vi "Measurement - PAE.vi"(7 "measure call context in":refnum<class "Measure Call Context.lvclass">, 8 "error in":errorcluster, 9 "RFmx Settings":T1={"RFmx Name"="5842_0", "RFmx Port"="", "Attenuation"={"Mode"=enum."Constant Attenuation", "Constant Attenuation"={"RFmx External Attenuation (dB)"=1.2}, "s2p File"={"RFmx S-Parameters Orientation"=24000, "RFmx Attenuation s2p File"=path ""}}} {"Attenuation"."s2p File"."RFmx S-Parameters Orientation" items=["Port1 Towards DUT"=24000, "Port2 Towards DUT"=24001]; "Attenuation"."Constant Attenuation"."RFmx External Attenuation (dB)" format="%.2f"}, 10 "RFSG Settings":T2={"RFSG Name"="5842_0", "RFSG Port"="", "Attenuation"={"Mode"=enum."Constant Attenuation", "Contant Attenuation"={"RFSG External Attenuation (dB)"=2.0}, "s2p File"={"RFSG S-parameters Orientation"=24000, "RFSG s2p File Path"=path ""}}} {"Attenuation"."s2p File"."RFSG S-parameters Orientation" items=["Port1 Towards DUT"=24000, "Port2 Towards DUT"=24001]; "Attenuation"."Contant Attenuation"."RFSG External Attenuation (dB)" format="%.2f"}, 11 "PAE Reference in":T3) -> (0 "error out":errorcluster, 3 "PAE Reference out":T3)   [LabVIEW 2023]
uses:
  <vilib>/niPAEML/Typedefs/Session Handle.ctl
  <vilib>/niPAEML/PAE Reference.lvclass
  Controls/RFSG Config - Compression.ctl
  Controls/RFmx Config - Compression.ctl
  <vilib>/Plug-In SDKs/Measurements/Measure Call Context/Measure Call Context.lvclass
  <instrlib>/niDCPower/nidcpower.llb/niDCPower Wait For Event - Event.ctl
  <vilib>/niPAEML/PAE Reference.lvclass/PAE Reference.ctl
  <vilib>/niPAEML/Accessors/Read RFSG Stimulus Mode.vi
  <vilib>/Analysis/baseanly.llb/Mean (DBL).vi
  <vilib>/RFmx/SpecAn/mx/RFmxSpecAn.llb/RFmxSpecAn TXP Fetch Measurement.vi
  <resource>/objmgr/RFmxSpecAn.rc
  <vilib>/niPAEML/PAE Measurement.lvlib
  <vilib>/Analysis/NI_AALBase.lvlib
panel:
  out "Current":dbl[](graph)
  out "Voltage":dbl[](graph)
  out "Pout":dbl[](graph)
  out "RF Input Sweep":dbl[](graph)
  out "Frequency Sweep":dbl[](graph)
  out "Power  Sweep Progress":dbl(slide)=1.0 scale=0.0..1.0
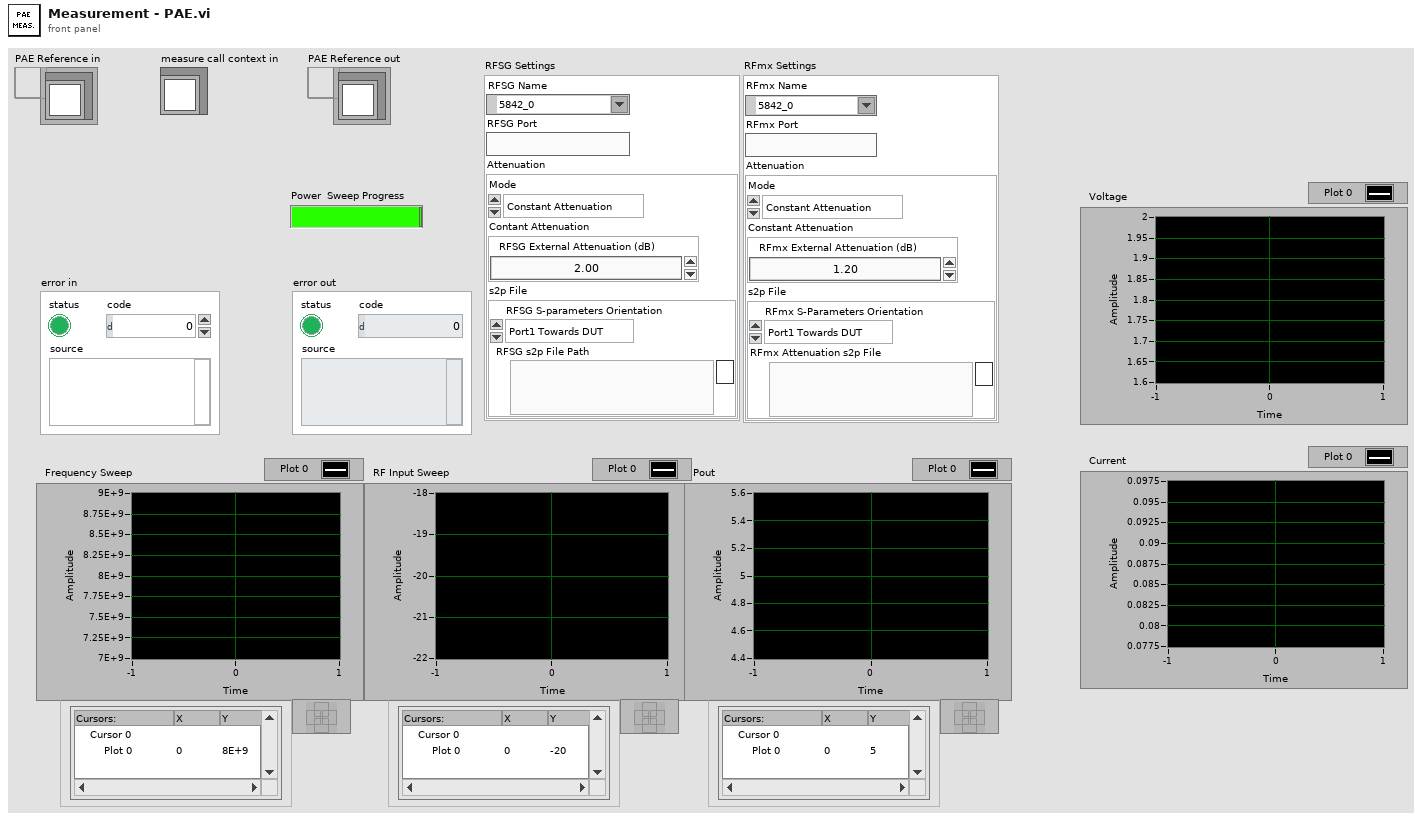
[diagram p1: front panel]
types:
  T1 = typedef "RFmx Config - Compression.ctl" = cluster{"RFmx Name":refnum<k15>, "RFmx Port":string, "Attenuation":cluster{"Mode":enum32{"<None>", "Constant Attenuation", "s2p File"}, "Constant Attenuation":cluster{"RFmx External Attenuation (dB)":dbl}, "s2p File":cluster{"RFmx S-Parameters Orientation":i32, "RFmx Attenuation s2p File":path}}}
  T2 = typedef "RFSG Config - Compression.ctl" = cluster{"RFSG Name":refnum<k15>, "RFSG Port":string, "Attenuation":cluster{"Mode":enum32{"<None>", "Constant Attenuation", "s2p File"}, "Contant Attenuation":cluster{"RFSG External Attenuation (dB)":dbl}, "s2p File":cluster{"RFSG S-parameters Orientation":i32, "RFSG s2p File Path":path}}}
  T3 = typedef "PAE Measurement.lvlib/PAE Reference.lvclass/Session Handle.ctl" = refnum<data-value>
  T4 = enum32{"<None>", "Constant Attenuation", "s2p File"}
  T5 = typedef "niDCPower Wait For Event - Event.ctl" = i32
  T6 = typedef "PAE Measurement.lvlib/PAE Reference.lvclass/RFSG Stimulus Mode.ctl" = enum16{"CW", "Pulsed CW"}
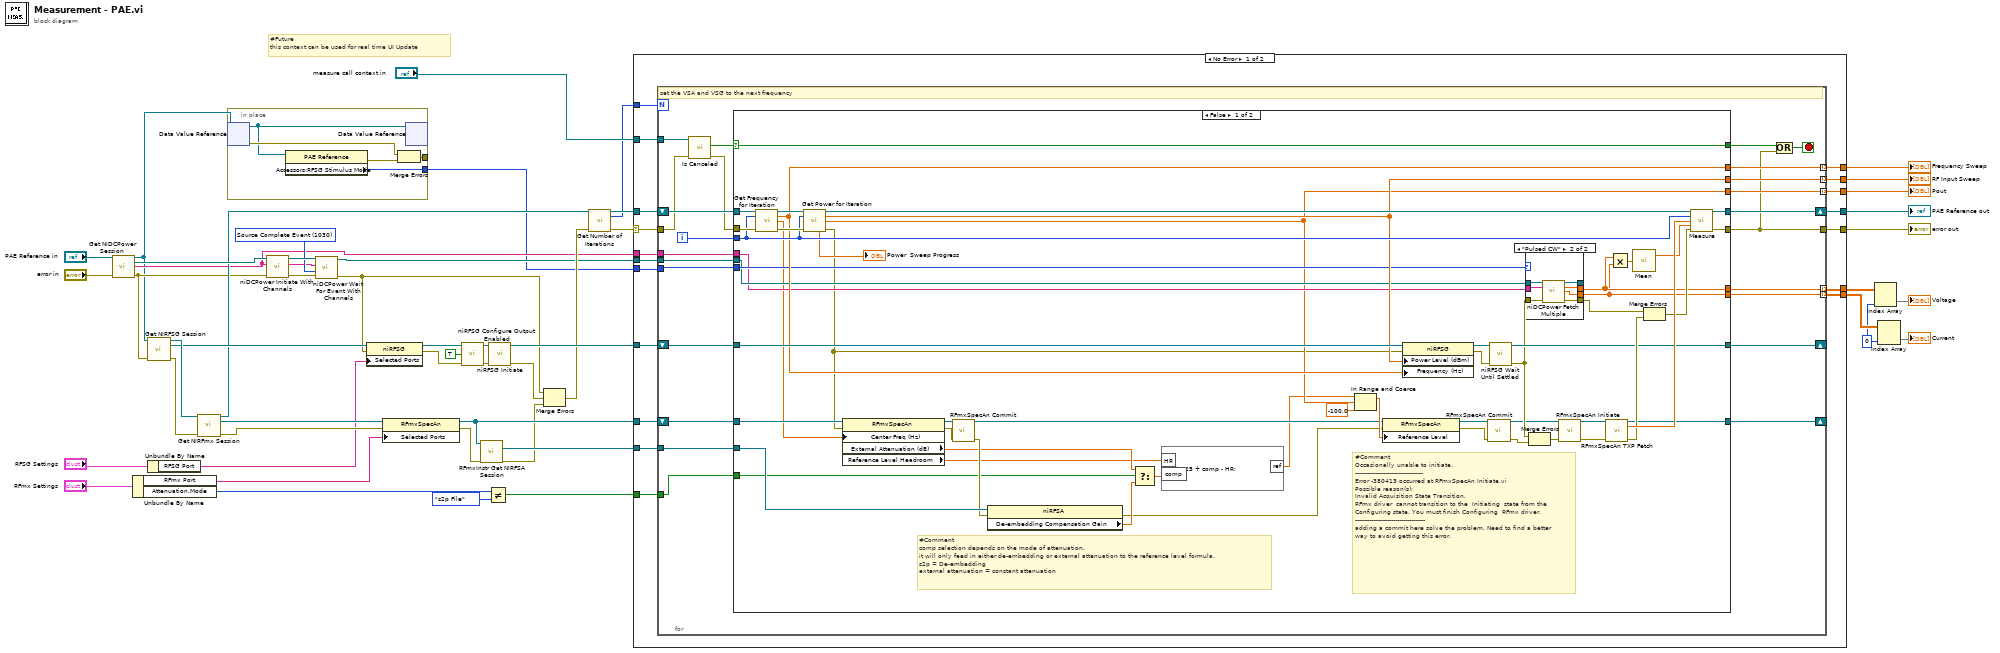
[diagram p0: block diagram]
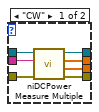
[diagram p2: hidden frame]
diagram:
  w13 = 0 ("disabled index (col)")
  w26 = T5 1030 items=["Source Complete Event"=1030, "Measure Complete Event"=1031, "Sequence Iteration Complete Event"=1032, "Sequence Engine Done Event"=1033, "Pulse Complete Event"=1051, "Ready For Pulse Trigger Event"=1052] ("event")
  # "#Future \nthis context can be used for real time UI Update"
  n1 = call <vilib>:"Get NIDCPower Session.vi"("PAE Reference In"="PAE Reference in", "error in"="error in") -> ("PAE Reference Out"=w11:T3, "NI DCPower Instrument Handle"=w25:refnum<k15>, "NI DCPower Channel Name"=w18:string, "error out"=w21:errorcluster)  [unwired: 10 in]
  n2 = Unbundle By Name("RFmx Settings") -> ("RFmx Port"=w32:string, "Attenuation.Mode"=w6:T4)
  n3 = Unbundle By Name("RFSG Settings") -> ("RFSG Port"=w33:string)
  n4 = call <vilib>:"Get NIRFSG Session.vi"("PAE Reference In"=w11, "error in"=w21) -> ("PAE Reference Out"=w44:T3, "NI RFSG Instrument Handle"=w39:refnum<k15>, "error out"=w37:errorcluster)  [unwired: 10 in, 1 out]
  n5 = call <vilib>:"Get NIRFmx Session.vi"("PAE Reference In"=w44, "error in"=w37) -> ("PAE Reference Out"=w24:T3, "NI RFmx Instrument Handle"=w41:refnum<k21>, "error out"=w40:errorcluster)  [unwired: 10 in, 1 out]
  n6 = in-place {
    in-place-border: [w52] -> _
    in-place-border: [w55] -> w12
    n7 = in-place-dvr #1(w11) -> (w54:refnum<class "PAE Reference.lvclass">, w56:errorcluster)
    n8 = property class="PAE Reference"(reference=w54) -> (error out=w53:errorcluster, "Accessors:RFSG Stimulus Mode"=w55:T6)  [unwired: 1 in, 1 out]
    n9 = Merge Errors(w56, w53) -> (w52:errorcluster)
    n10 = in-place-dvr #1(w54) -> ()  [unwired: 2 out]
  }
  n11 = call <instrlib>:"niDCPower Initiate With Channels.vi"("error in (no error)"=w21, "channel name"=w18, "instrument handle"=w25) -> ("error out"=w27:errorcluster, "instrument handle out"=w28:refnum<k15>)  [unwired: 7 in]
  n12 = call <instrlib>:"niDCPower Wait For Event With Channels.vi"("error in (no error)"=w27, "event"=w26, "channel name"=w18, "instrument handle"=w28) -> ("error out"=w20:errorcluster, "instrument handle out"=w19:refnum<k15>)  [unwired: 6 in]
  n13 = property class="niRFSG"(reference=w39, error in=w20, "Selected Ports"=w33) -> (reference out=w38:refnum<k15>, error out=w36:errorcluster)
  n14 = property class="RFmxSpecAn"(reference=w41, error in=w40, "Selected Ports"=w32) -> (reference out=w10:refnum<k21>, error out=w9:errorcluster)
  n15 = call <instrlib>:"niRFSG Configure Output Enabled.vi"("instrument handle"=w38, "output enabled"=TRUE ("output enable"), "error in"=w36) -> ("instrument handle out"=w46:refnum<k15>, "error out"=w47:errorcluster)  [unwired: 11 out]
  n16 = call <vilib>:"RFmxInstr Get NIRFSA Session.vi"("Instrument Handle In"=w10, "error in (no error)"=w9) -> ("NI RFSA Session"=w8:refnum<k15>, "error out"=w7:errorcluster)  [unwired: 11 in, 1 out]
  n17 = Not Equal?(x=w6, y=T4."s2p File") -> (x != y?=w4:bool)
  n18 = call <instrlib>:"niRFSG Initiate.vi"("instrument handle"=w46, "error in"=w47) -> ("instrument handle out"=w49:refnum<k15>, "error out"=w48:errorcluster)  [unwired: 12 out]
  n19 = Merge Errors(w20, w48, w7) -> (w43:errorcluster)
  n20 = call <vilib>:"Get Number of Iterations.vi"("PAE Reference In"=w24, "error in"=w43) -> ("PAE Reference Out"=w42:T3, "Total Number of Iterations"=w1:i32, "error out"=w2:errorcluster)  [unwired: 9 in, 2 out]
  n21 = case shown="No Error" w2 {
    selector: w2 -> [w60 w173]
    tunnel: [w74 w173] -> w51
    tunnel: [w73 w172] -> w50
    tunnel: w1 -> [w72 _]
    tunnel: w49 -> [w71 _]
    tunnel: w42 -> [w70 w172]
    tunnel: w10 -> [w69 _]
    tunnel: [w68 _] -> w31
    tunnel: [w67 _] -> w30
    tunnel: [w66 _] -> w29
    tunnel: w19 -> [w65 _]
    tunnel: w18 -> [w64 _]
    tunnel: [w63 _] -> w17
    tunnel: [w62 _] -> w16
    tunnel: w12 -> [w61 _]
    tunnel: w8 -> [w59 _]
    tunnel: w4 -> [w58 _]
    tunnel: "measure call context in" -> [w57 _]
    frame No Error {
      n22 = for {
        N: w72 -> [_]
        shift-right: [w92] -> _
        shift-left: w69 -> [w84]
        shift-right: [w91] -> _
        shift-left: w71 -> [w98]
        shift-right: [w95] -> w73
        shift-left: w70 -> [w97]
        tunnel: w60 -> [w76]
        tunnel: [w79] -> w74
        tunnel: [w94] -> w67 mode=indexing
        tunnel: [w85] -> w66 mode=indexing
        tunnel: [w93] -> w68 mode=indexing
        tunnel: w61 -> [w90]
        tunnel: w65 -> [w89]
        tunnel: w64 -> [w88]
        tunnel: [w87] -> w62 mode=indexing
        tunnel: [w86] -> w63 mode=indexing
        tunnel: w59 -> [w83]
        tunnel: w58 -> [w82]
        tunnel: w57 -> [w81]
        i -> [w96]
        stop <- w80 stop-if-true
        # "set the VSA and VSG to the next frequency"
        n23 = call <vilib>:"Is Canceled.vi"("error in"=w76, "measure call context in"=w81) -> ("error out"=w75:errorcluster, "is canceled?"=w77:bool)  [unwired: 7 in, 1 out]
        n24 = case shown="False" w77 {
          selector: w77 -> [w99 w171]
          tunnel: w98 -> [w152 w168]
          tunnel: w97 -> [w150 w170]
          tunnel: w75 -> [w144 w169]
          tunnel: w96 -> [w142 _]
          tunnel: [w136 w170] -> w95
          tunnel: [w135 _] -> w94
          tunnel: [w134 _] -> w93
          tunnel: [w133 w167] -> w92
          tunnel: [w132 w168] -> w91
          tunnel: w90 -> [w129 _]
          tunnel: w89 -> [w128 _]
          tunnel: w88 -> [w127 _]
          tunnel: [w125 _] -> w87
          tunnel: [w124 _] -> w86
          tunnel: [w123 _] -> w85
          tunnel: w84 -> [w120 w167]
          tunnel: w83 -> [w113 _]
          tunnel: w82 -> [w109 _]
          tunnel: [w100 w169] -> w79
          tunnel: [w99 w171] -> w78
          frame False {
            # "#Comment\nOccasionally unable to initiate. \n----------------------------------\nError -380413 occurred at RFmxSpecAn Initiate.vi\nPossible reason(s):\nInvalid Acquisition State Transition.\nRFmx driver  cannot transition to the  Initiating  state from the Configuring state. You must finish Configuring  RFmx driver.\n-----------------------------------\nadding a commit here solve the problem. Need to find a better way to avoid getting this error."
            # "#Comment\ncomp selection depends on the mode of attenuation.\nit will only feed in either de-embedding or external attenuation to the reference level formula.\ns2p = De-embedding \nexternal attenuation = constant attenuation"
            n25 = call <vilib>:"Get Frequency for Iteration.vi"("PAE Reference In"=w150, "Loop Iteration Index"=w142, "error in"=w144) -> ("PAE Reference Out"=w151:T3, "NI RFSG Frequency (Hz)"=w134:dbl, "NI RFmx Frequency (Hz)"=w119:dbl, "error out"=w143:errorcluster)  [unwired: 7 in, 2 out]
            n26 = call <vilib>:"Get Power for Iteration.vi"("PAE Reference In"=w151, "Loop Iteration Index"=w142, "error in"=w143) -> ("PAE Reference Out"=w139:T3, "NI RFSG Power (dBm)"=w135:dbl, "NI RFmx Power (dBm)"=w123:dbl, "Power Iteration Fraction"=→"Power  Sweep Progress":dbl, "error out"=w118:errorcluster)  [unwired: 7 in, 1 out]
            n27 = property class="RFmxSpecAn"(reference=w120, error in=w118, "Center Freq (Hz)"=w119) -> (reference out=w117:refnum<k21>, error out=w115:errorcluster, "External Attenuation (dB)"=w106:dbl, "Reference Level Headroom"=w105:dbl)
            n28 = call <vilib>:"RFmxSpecAn Commit.vi"("Instrument Handle In"=w117, "error in (no error)"=w115) -> ("Instrument Handle Out"=w116:refnum<k21>, "error out"=w112:errorcluster)  [unwired: 12 in]
            n29 = property class="niRFSA"(reference=w113, error in=w112) -> (error out=w107:errorcluster, "De-embedding Compensation Gain"=w108:dbl)  [unwired: 1 out]
            n30 = Select(t=w106, s=w109, f=w108) -> (s? t:f=w110:dbl)
            n31 = formula code="ref = 25 + comp - HR;"("HR"=w105, "comp"=w110) -> ("ref"=w111:dbl)
            n32 = In Range and Coerce(upper limit=w111, x=w123, lower limit=-100.0) -> (coerced(x)=w122:dbl)  [unwired: 1 out]
            n33 = property class="RFmxSpecAn"(reference=w116, error in=w107, "Reference Level"=w122) -> (reference out=w104:refnum<k21>, error out=w101:errorcluster)
            n34 = property class="niRFSG"(reference=w152, error in=w118, "Power Level (dBm)"=w135, "Frequency (Hz)"=w134) -> (reference out=w147:refnum<k15>, error out=w146:errorcluster)
            n35 = call <vilib>:"RFmxSpecAn Commit.vi"("Instrument Handle In"=w104, "error in (no error)"=w101) -> ("Instrument Handle Out"=w103:refnum<k21>, "error out"=w102:errorcluster)  [unwired: 12 in]
            n36 = call <instrlib>:"niRFSG Wait Until Settled.vi"("instrument handle"=w147, "error in"=w146) -> ("instrument handle out"=w132:refnum<k15>, "error out"=w121:errorcluster)  [unwired: 12 in]
            n37 = case shown="\"Pulsed CW\"" w129 {
              tunnel: [w159 w162] -> _
              tunnel: w127 -> [w158 w163]
              tunnel: [w157 w161] -> w125
              tunnel: [w156 w160] -> w124
              tunnel: w128 -> [w155 w164]
              tunnel: w121 -> [w154 w166]
              tunnel: [w153 w165] -> w126
              frame "CW" {
                n38 = call <instrlib>:"niDCPower Measure Multiple.vi"("error in (no error)"=w154, "channel name"=w158, "instrument handle"=w155) -> ("error out"=w153:errorcluster, "current measurements"=w156:dbl[], "voltage measurements"=w157:dbl[], "instrument handle out"=w159:refnum<k15>)  [unwired: 5 in]
              }
              frame "Pulsed CW" {
                n39 = call <instrlib>:"niDCPower Fetch Multiple.vi"("instrument handle"=w164, "channel name"=w163, "error in (no error)"=w166) -> ("instrument handle out"=w162:refnum<k15>, "voltage measurements"=w161:dbl[], "current measurements"=w160:dbl[], "error out"=w165:errorcluster)  [unwired: 7 in, 2 out]
              }
            }
            n40 = Merge Errors(w121, w102) -> (w138:errorcluster)
            n41 = call <vilib>:"RFmxSpecAn Initiate.vi"("Instrument Handle In"=w103, "error in (no error)"=w138) -> ("Instrument Handle Out"=w148:refnum<k21>, "error out"=w149:errorcluster)  [unwired: 11 in, 1 out]
            n42 = call-poly <vilib>:"RFmxSpecAn TXP Fetch.vi"("Instrument Handle In"=w148, "error in (no error)"=w149) -> ("Instrument Handle Out"=w133:refnum<k21>, "Average Mean Power (dBm)"=w145:dbl, "error out"=w140:errorcluster)  [unwired: 8 in, 3 out]
            n43 = Multiply(x=w125, y=w124) -> (x*y=w131:dbl[])
            n44 = call-poly <vilib>:"Mean.vi"("X"=w131) -> ("mean"=w130:dbl)  [unwired: 1 out]
            n45 = Merge Errors(w126, w140) -> (w137:errorcluster)
            n46 = call <vilib>:"Measure.vi"("PAE Reference In"=w139, "Loop Iteration Index"=w142, "Measured RF Power"=w145, "Measured DC Power"=w130, "error in"=w137) -> ("PAE Reference Out"=w136:T3, "error out"=w100:errorcluster)  [unwired: 9 in]
          }
          frame True {
            # "Canceled"
          }
        }
        n47 = Compound Arithmetic op=OR(w78, w79) -> (w80:bool)
      }
    }
    frame Error {
    }
  }
  "error out" <- w51
  "PAE Reference out" <- w50
  "Frequency Sweep" <- w31
  "Pout" <- w29
  "RF Input Sweep" <- w30
  n48 = Index Array(array=w16, index (col)=w13) -> (element=→"Voltage":dbl[])  [unwired: 1 in]
  n49 = Index Array(array=w17, index (col)=w13) -> (element=→"Current":dbl[])  [unwired: 1 in]
